vi "Put Blob.vi"(6 "Blob Content":string, 7 "Blob type":T1, 8 "error in (no error)":errorcluster, 9 "Blob":string, 10 "Container":string, 11 "Azure Session in":refnum<class "Session.lvclass">) -> (0 "error out":errorcluster, 3 "Azure Session out":refnum<class "Session.lvclass">)   [LabVIEW 2015, in "NI_Azure_Blob.lvlib"]
doc: "Creates a new blob or replaces an existing blob within a container."
uses:
  NI_Azure_Blob.lvlib
  Core/Session/Session.lvclass
  Blob Type.ctl
  Core/Name Value Pair.ctl
  Core/Session/Session.lvclass/Session.ctl
  Core/Session/Write Request body.vi
  Core/Session/Write Request Headers.vi
  Core/Session/Write HTTP Verb.vi
  Core/Session/Write URL Suffix.vi
  Core/NI_Azure_Core.lvlib
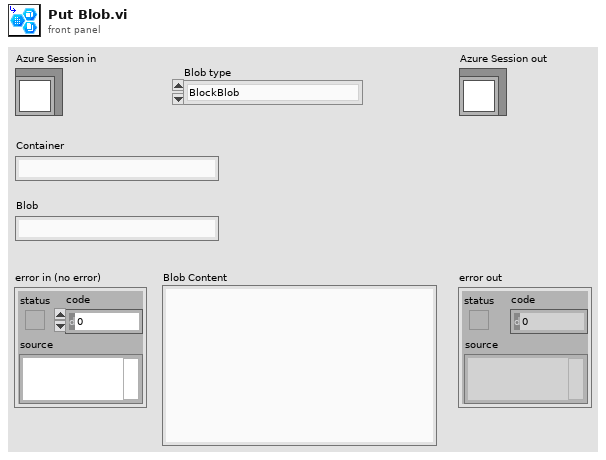
[diagram p1: front panel]
types:
  T1 = typedef "NI_Azure_Blob.lvlib/Blob Type.ctl" = enum16{"BlockBlob", "PageBlob", "AppendBlob"}
  T2 = typedef "NI_Azure_Core.lvlib/Name Value Pair.ctl" = cluster{"name":string, "value":string}
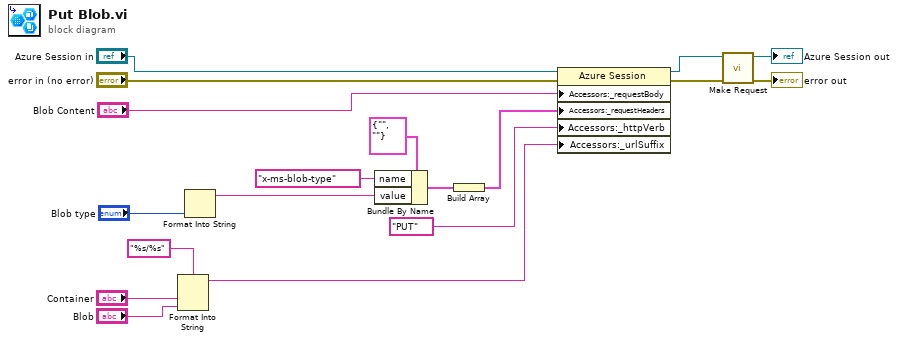
[diagram p0: block diagram]
diagram:
  n1 = Format Into String(format string="%s/%s", "Container", "Blob") -> (resulting string=w1:string)  [unwired: 2 in, 1 out]
  n2 = Format Into String("Blob type") -> (resulting string=w9:string)  [unwired: 3 in, 1 out]
  n3 = Bundle By Name(cluster=T2 {"name"="", "value"=""} ("Name Value Pair"), "name"="x-ms-blob-type" ("header"), "value"=w9) -> (w11:T2)
  n4 = Build Array(w11) -> (w3:T2[])
  n5 = property class="Azure Session"(reference="Azure Session in", error in="error in (no error)", "Accessors:_requestBody"="Blob Content", "Accessors:_requestHeaders"=w3, "Accessors:_httpVerb"="PUT" ("HTTP-Verb"), "Accessors:_urlSuffix"=w1) -> (reference out=w7:refnum<class "Session.lvclass">, error out=w5:errorcluster)
  n6 = call "Make Request.vi"("error in (no error)"=w5, "Session in"=w7) -> ("error out"=→"error out":errorcluster, "Session out"=→"Azure Session out":refnum<class "Session.lvclass">)  [unwired: 7 in, 1 out]
